vi "convert Jl functions enum to string.vi"(8 "error in (no error)":errorcluster, 11 "fun2call":T1) -> (0 "error out":errorcluster, 3 "String out":string)   [LabVIEW 2018, in "LV-Julia_ZMQ-Roundtrip_lib.lvlib"]
uses:
  LV-Julia_ZMQ-Roundtrip_lib.lvlib
  Julia functions enum.ctl
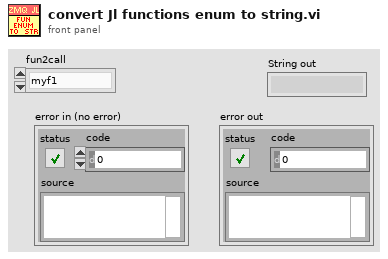
[diagram p1: front panel]
types:
  T1 = typedef "LV-Julia_ZMQ-Roundtrip_lib.lvlib/Julia functions enum.ctl" = enum16{"myf1", "myf2", "myf3", "bin2num"}
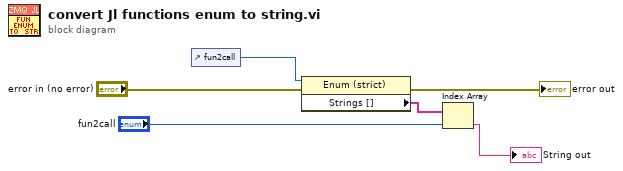
[diagram p0: block diagram]
diagram:
  n1 = control-ref of="fun2call"() -> (w1:refnum<vi>)
  n2 = property on="Property Node" class="Enum (strict)"(reference=w1, error in="error in (no error)") -> (error out=→"error out":errorcluster, "Strings []"=w2:string[])  [unwired: 1 out]
  n3 = Index Array(array=w2, index="fun2call") -> (element=→"String out":string)
